vi "CheckGameBoard.vi"(8 "error in (no error)":errorcluster, 11 "Board in":T1[][](array[typedef])) -> (0 "error out":errorcluster, 3 "Board out":T1[][](array[typedef]))   [LabVIEW 2020]
uses:
  TypeDef/tiles-key-trunct.ctl
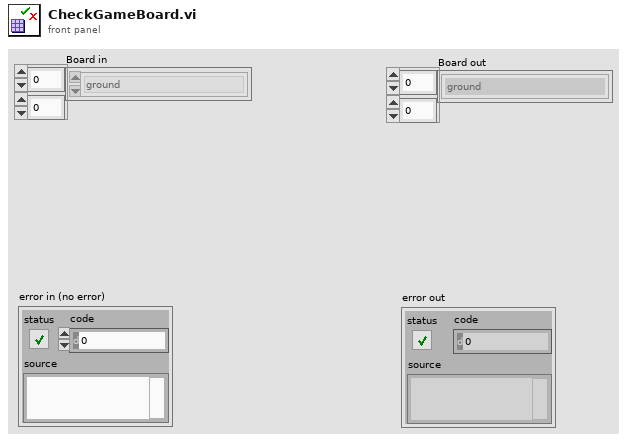
[diagram p1: front panel]
types:
  T1 = typedef "tiles-key-trunct.ctl" = enum16{"ground", "wall", "head (right)", "head (up)", "head (left)", "head (down)", "L-turn (right-up)", "L-turn (up-left)", "L-turn (left-down)", "L-turn (down-right)", "body (right)", "body (up)", "body (left)", "body (down)", "R-turn (right-down)", "R-turn (up-right)", "R-turn (left-up)", "R-turn (down-left)", "tail (right)", "tail (up)", "tail (left)", "tail (down)"}
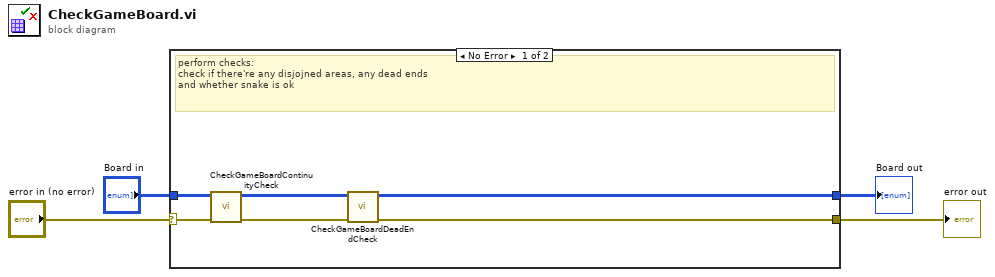
[diagram p0: block diagram]
diagram:
  n1 = case shown="No Error" "error in (no error)" {
    selector: "error in (no error)" -> [w10 w12]
    tunnel: "Board in" -> [w7 w11]
    tunnel: [w5 w11] -> w2
    tunnel: [w8 w12] -> w1
    frame No Error {
      # "perform checks:\ncheck if there're any disjojned areas, any dead ends \nand whether snake is ok"
      n2 = call "CheckGameBoardContinuityCheck.vi"("error in (no error)"=w10, "Board in"=w7) -> ("error out"=w9:errorcluster, "Board out"=w6:T1[][])  [unwired: 6 in, 2 out]
      n3 = call "CheckGameBoardDeadEndCheck.vi"("error in (no error)"=w9, "Board in"=w6) -> ("error out"=w8:errorcluster, "Board out"=w5:T1[][])  [unwired: 7 in, 1 out]
    }
    frame Error {
    }
  }
  "Board out" <- w2
  "error out" <- w1
